vi "rethinkdb_connect.vi"(6 "ms timeout (10000)":i32=10000, 8 "error in (no error)":errorcluster, 9 "auth":T1={"user"="user", "password"="rOprNGfwEbeRWgbNEkqO"}, 10 "port (28015)":u16=28015, 11 "host (\"localhost\")":string="localhost") -> (0 "error out":errorcluster, 2 "server_final_json":string, 3 "rethinkdb":refnum<k5>)   [LabVIEW 2017]
uses:
  msg/rethinkdb_msg_connect_auth.ctl
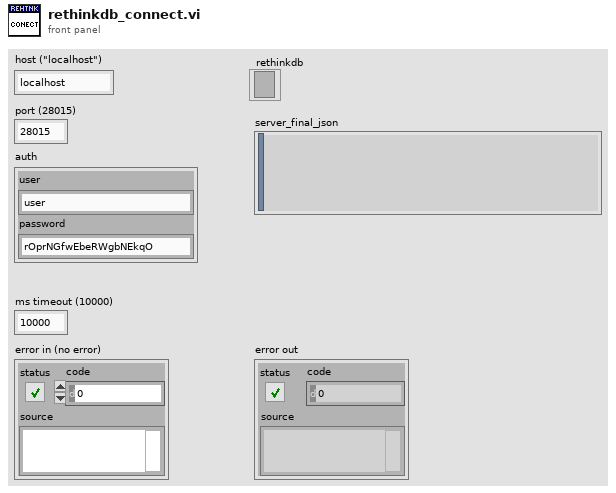
[diagram p1: front panel]
types:
  T1 = typedef "rethinkdb_msg_connect_auth.ctl" = cluster{"user":string, "password":string}
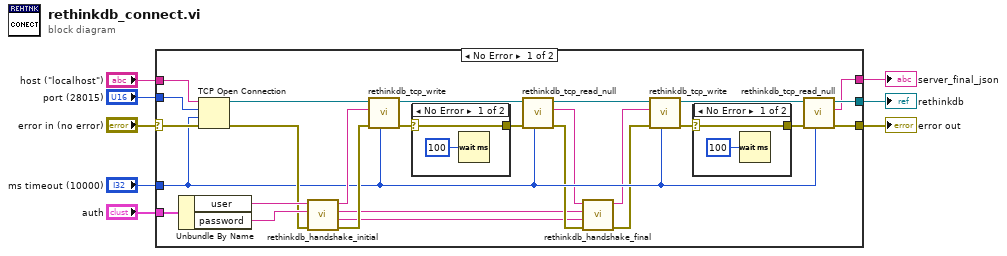
[diagram p0: block diagram]
diagram:
  n1 = case shown="No Error" "error in (no error)" {
    selector: "error in (no error)" -> [w35 w42]
    tunnel: "host (\"localhost\")" -> [w34 _]
    tunnel: "port (28015)" -> [w33 _]
    tunnel: "ms timeout (10000)" -> [w23 _]
    tunnel: [w12 w42] -> w4
    tunnel: [w13 _] -> w3
    tunnel: "auth" -> [w32 _]
    tunnel: [w9 _] -> w1
    frame No Error {
      n2 = Unbundle By Name(w32) -> ("user"=w31:string, "password"=w30:string)
      n3 = TCP Open Connection(address=w34, remote port or service name=w33, timeout ms (60000)=w23, error in (no error)=w35) -> (connection ID=w28:refnum<k5>, error out=w27:errorcluster)  [unwired: 1 in]
      n4 = call "rethinkdb_handshake_initial.vi"("error in (no error)"=w27, "password"=w30, "user"=w31) -> ("error out"=w26:errorcluster, "client_first_message"=w10:string, "dup password"=w11:string, "initial_message"=w25:string)  [unwired: 5 in]
      n5 = call "rethinkdb_tcp_write.vi"("timeout ms (10000)"=w23, "error in (no error)"=w26, "data in"=w25, "rethinkdb in"=w28) -> ("error out"=w17:errorcluster, "rethinkdb out"=w29:refnum<k5>)  [unwired: 5 in, 1 out]
      n6 = case shown="No Error" w17 {
        selector: w17 -> [w39 w41]
        tunnel: [w39 w41] -> w18
        frame No Error {
          n7 = Wait (ms)(milliseconds to wait=u32 100) -> ()  [unwired: 1 out]
        }
        frame Error {
        }
      }
      n8 = call "rethinkdb_tcp_read_null.vi"("timeout ms (10000)"=w23, "error in (no error)"=w18, "rethinkdb in"=w29) -> ("error out"=w21:errorcluster, "data out"=w19:string, "rethinkdb out"=w22:refnum<k5>)  [unwired: 6 in]
      n9 = call "rethinkdb_handshake_final.vi"("error in (no error)"=w21, "client_first_message"=w10, "password"=w11, "server_response (json)"=w19) -> ("error out"=w20:errorcluster, "authentication_request"=w16:string)  [unwired: 6 in]
      n10 = call "rethinkdb_tcp_write.vi"("timeout ms (10000)"=w23, "error in (no error)"=w20, "data in"=w16, "rethinkdb in"=w22) -> ("error out"=w14:errorcluster, "rethinkdb out"=w24:refnum<k5>)  [unwired: 5 in, 1 out]
      n11 = case shown="No Error" w14 {
        selector: w14 -> [w36 w38]
        tunnel: [w36 w38] -> w15
        frame No Error {
          n12 = Wait (ms)(milliseconds to wait=u32 100) -> ()  [unwired: 1 out]
        }
        frame Error {
        }
      }
      n13 = call "rethinkdb_tcp_read_null.vi"("timeout ms (10000)"=w23, "error in (no error)"=w15, "rethinkdb in"=w24) -> ("error out"=w12:errorcluster, "data out"=w9:string, "rethinkdb out"=w13:refnum<k5>)  [unwired: 6 in]
    }
    frame Error {
    }
  }
  "error out" <- w4
  "rethinkdb" <- w3
  "server_final_json" <- w1
